vi "AH2500.RW.vi"(8 "error in (no error)":errorcluster, 10 "write buffer":string, 11 "VISA Refnum in":refnum<visa-resource-name>) -> (0 "error out":errorcluster, 2 "read buffer":string, 3 "VISA Refnum out":refnum<visa-resource-name>)   [LabVIEW 2019, in "Inst.AH2500.lvclass"]
uses:
  Inst.AH2500.lvclass
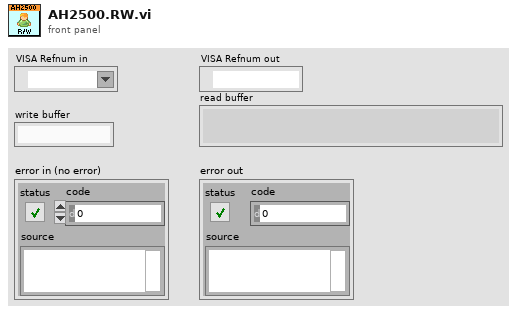
[diagram p1: front panel]
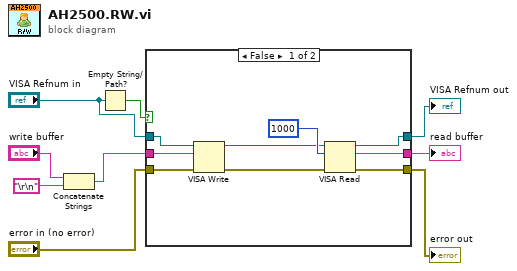
[diagram p0: block diagram]
diagram:
  n1 = Concatenate Strings("write buffer", "\r\n") -> (w1:string)
  n2 = Empty String/Path?(string/path="VISA Refnum in") -> (empty?=w4:bool)
  n3 = case shown="False" w4 {
    tunnel: [w18 w19] -> w9
    tunnel: [w17 w20] -> w8
    tunnel: [w16 w21] -> w7
    tunnel: w1 -> [w15 w19]
    tunnel: "error in (no error)" -> [w14 w20]
    tunnel: "VISA Refnum in" -> [w13 w21]
    frame False {
      n4 = VISA Write(VISA resource name=w13, write buffer=w15, error in (no error)=w14) -> (VISA resource name out=w10:refnum<visa-resource-name>, error out=w12:errorcluster)  [unwired: 1 out]
      n5 = VISA Read(VISA resource name=w10, byte count=u32 1000, error in (no error)=w12) -> (VISA resource name out=w16:refnum<visa-resource-name>, read buffer=w18:string, error out=w17:errorcluster)  [unwired: 1 out]
    }
    frame True {
    }
  }
  "read buffer" <- w9
  "error out" <- w8
  "VISA Refnum out" <- w7
